vi "Generic command handler.vi"(8 "error in (no error)":errorcluster, 10 "Message in":refnum<class "GenericMessage.lvclass">, 11 "Test_ExampleClassA in":refnum<class "Test_ExampleClassA.lvclass">) -> (0 "error out":errorcluster, 2 "value":string, 3 "Test_ExampleClassA out":refnum<class "Test_ExampleClassA.lvclass">)   [LabVIEW 2012, in "Test_ExampleClassA.lvclass"]
doc: "Handles the generic internal command \"proceed\", that is used to go from test to test."
uses:
  Test_ExampleClassA.lvclass
  GenericMessage/GenericMessage.lvclass
  MurmexTest/MurmexTest.lvclass
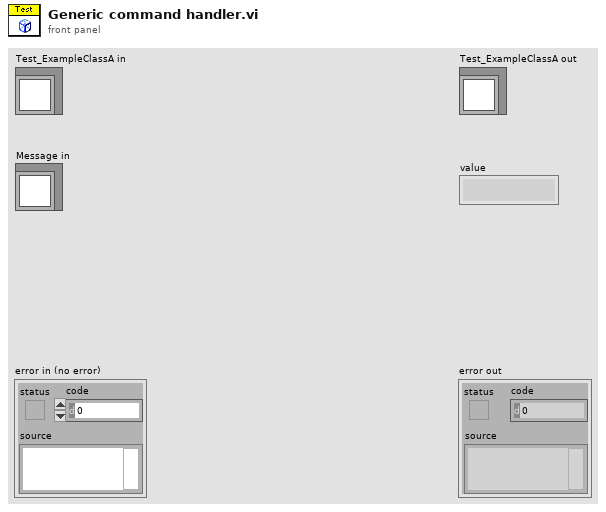
[diagram p1: front panel]
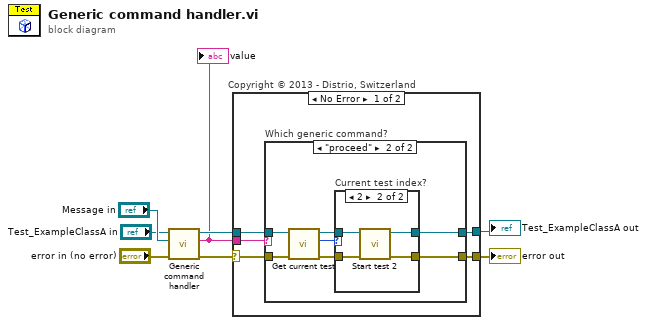
[diagram p0: block diagram]
diagram:
  n1 = call-parent "Generic command handler.vi"("error in (no error)"="error in (no error)", "Message in"="Message in", "MurmexTest in"="Test_ExampleClassA in") -> ("error out"=w5:errorcluster, "value"=w1:string, "MurmexTest out"=w4:refnum<class "Test_ExampleClassA.lvclass">)  [unwired: 6 in]
  "value" <- w1
  n2 = case "Copyright © 2013 - Distrio, Switzerland" shown="No Error" w5 {
    selector: w5 -> [w11 w29]
    tunnel: w4 -> [w12 w30]
    tunnel: [w10 w30] -> w3
    tunnel: [w13 w29] -> w2
    tunnel: w1 -> [w9 _]
    frame No Error {
      n3 = case "Which generic command?" shown="\"proceed\"" w9 {
        tunnel: [w14 w22] -> w13
        tunnel: w12 -> [w15 w20]
        tunnel: w11 -> [w14 w17]
        tunnel: [w15 w16] -> w10
        frame Default {
        }
        frame "proceed" {
          n4 = call "Get current test.vi"("error in (no error)"=w17, "MurmexTest in"=w20) -> ("error out"=w18:errorcluster, "test index"=w21:i32, "MurmexTest out"=w19:refnum<class "Test_ExampleClassA.lvclass">)  [unwired: 7 in]
          n5 = case "Current test index?" shown="2" w21 {
            tunnel: w18 -> [w23 w28]
            tunnel: w19 -> [w24 w27]
            tunnel: [w23 w26] -> w22
            tunnel: [w24 w25] -> w16
            frame Default {
            }
            frame 2 {
              n6 = call "Start test 2.vi"("error in (no error)"=w28, "Test_ExampleClassA in"=w27) -> ("error out"=w26:errorcluster, "Test_ExampleClassA out"=w25:refnum<class "Test_ExampleClassA.lvclass">)  [unwired: 8 in]
            }
          }
        }
      }
    }
    frame Error {
    }
  }
  "error out" <- w2
  "Test_ExampleClassA out" <- w3
